vi "MRC Alert Set Alert Active.vi"(8 "error in (no error)":errorcluster, 10 "active":u8, 11 "handle":i64) -> (0 "error out":errorcluster)   [LabVIEW 2026, in "MrcLib.lvlib"]
doc: "MRC_Status MRC_CALLCONV MRC_Alert_SetAlertActive(MRC_AlertHandle handle,\n MRC_Bool active);"
uses:
  MrcLib.lvlib
  MrcLib.dll
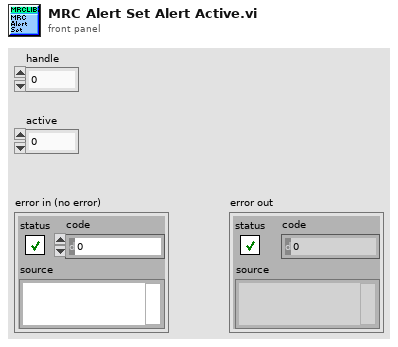
[diagram p1: front panel]
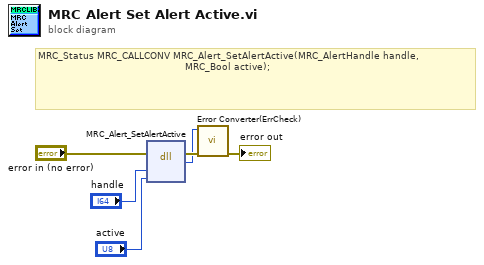
[diagram p0: block diagram]
diagram:
  # "MRC_Status MRC_CALLCONV MRC_Alert_SetAlertActive(MRC_AlertHandle handle,\n                                                 MRC_Bool active);"
  n1 = dll-call lib="MrcLib.*" fn="MRC_Alert_SetAlertActive"(error in="error in (no error)", "handle"="handle", "active"="active") -> (error out=w2:errorcluster, w1:i32)  [unwired: 4 in, 1 out]
  n2 = call <vilib>:"Error Converter(ErrCheck).vi"("error in (no error)"=w2, "status"=w1) -> ("error out"=→"error out":errorcluster)  [unwired: 9 in]
